vi "HTTP PUT File.vi"(8 "error in (no error)":errorcluster, 9 "file":path, 10 "Endpoint":string, 11 "REST_Client in":refnum<class "REST_Client.lvclass">) -> (0 "error out":errorcluster, 1 "body":string, 2 "headers":string, 3 "REST_Client out":refnum<class "REST_Client.lvclass">)   [LabVIEW 2020, in "REST_Client.lvclass"]
uses:
  REST_Client.lvclass
  <vilib>/httpClient/LabVIEWHTTPClient.lvlib
  <vilib>/httpClient/PUTFile.vi
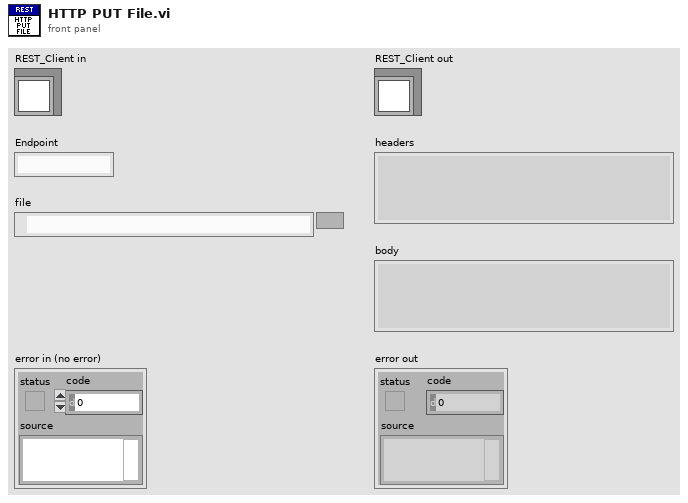
[diagram p1: front panel]
types:
  T1 = typedef "LabVIEWHTTPClient.lvlib/ClientHandle.ctl" = refnum<k1>
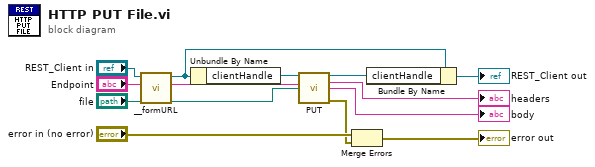
[diagram p0: block diagram]
diagram:
  n1 = call "__formURL.vi"("endPoint"="Endpoint", "REST_Client in"="REST_Client in") -> ("URL"=w11:string, "REST_Client out"=w9:refnum<class "REST_Client.lvclass">)  [unwired: 8 in]
  n2 = Unbundle By Name(w9) -> ("clientHandle"=w12:T1)
  n3 = call-poly <vilib>:"PUT.vi"("client handle"=w12, "url"=w11, "file"="file") -> ("client handle out"=w8:T1, "headers"=→"headers":string, "body"=→"body":string, "error out"=w3:errorcluster)  [unwired: 9 in]
  n4 = Merge Errors("error in (no error)", w3) -> (→"error out":errorcluster)
  n5 = Bundle By Name(cluster=w9, "clientHandle"=w8) -> (→"REST_Client out":refnum<class "REST_Client.lvclass">)
